vi "Arduino_DigitalRead1.vi"() -> ()   [LabVIEW 2019]
uses:
  <vilib>/LabVIEW Interface for Arduino/Type Defs/Pin Mode.ctl
  <vilib>/LabVIEW Interface for Arduino/Type Defs/Board Type.ctl
  <vilib>/LabVIEW Interface for Arduino/Type Defs/Connection Type.ctl
  <vilib>/LabVIEW Interface for Arduino/LabVIEW Interface for Arduino.lvlib
panel:
  in  "Connection Type (USB/Serial)":T1
  in  "Bytes Per Packet (15)":u32=15
  in  "Board Type (Uno)":T2
  in  "Baud Rate (115200)":u32=115200
  in  "VISA resource":refnum<visa-resource-name>
  out "Value":u8
  out "error close":errorcluster
  out "error read":errorcluster
  in  "stop":bool
  out "error init":errorcluster
  out "error o/i":errorcluster
  in  "Pin Mode (Input)":T3
  in  "Digital I/O Pin":u8
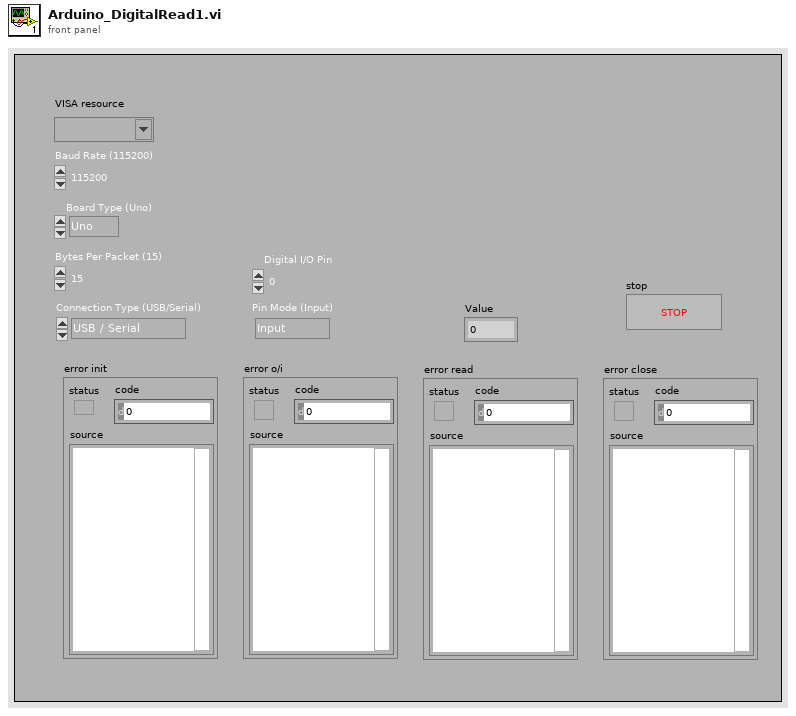
[diagram p1: front panel]
types:
  T1 = typedef "LabVIEW Interface for Arduino.lvlib/Connection Type.ctl" = enum8{"USB / Serial", "XBEE", "BlueSmirf (Bluetooth)"}
  T2 = typedef "LabVIEW Interface for Arduino.lvlib/Board Type.ctl" = enum16{"Uno", "Dimuelanove w/Atmega 328", "Mega 2560"}
  T3 = typedef "LabVIEW Interface for Arduino.lvlib/Pin Mode.ctl" = enum8{"Input", "Output"}
  T4 = typedef "LabVIEW Interface for Arduino.lvlib/Arduino Resource.ctl" = cluster{"VISA resource":refnum<visa-resource-name>, "Board Type":T2, "Connection Type":enum8{"USB / Serial"}, "Bytes Per Packet (15)":u8}
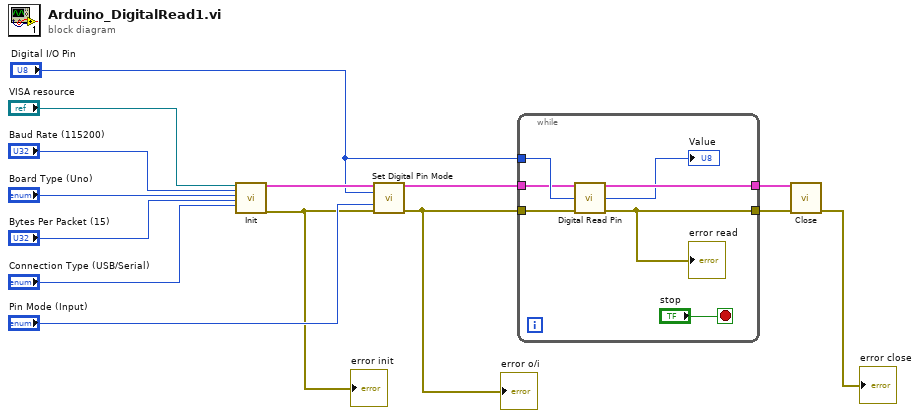
[diagram p0: block diagram]
diagram:
  n1 = call <vilib>:"Init.vi"("VISA resource"="VISA resource", "Baud Rate (115200)"="Baud Rate (115200)", "Board Type (Uno)"="Board Type (Uno)", "Bytes Per Packet (15)"="Bytes Per Packet (15)", "Connection Type (USB/Serial)"="Connection Type (USB/Serial)") -> ("Arduino Resource"=w13:T4, "error out"=w12:errorcluster)  [unwired: 13 in]
  "error init" <- w12
  n2 = call <vilib>:"Set Digital Pin Mode.vi"("Arduino Resource"=w13, "Digital I/O Pin"="Digital I/O Pin", "Pin Mode (Input)"="Pin Mode (Input)", "error in"=w12) -> ("Arduino Resource"=w9:T4, "error out"=w10:errorcluster)  [unwired: 10 in]
  "error o/i" <- w10
  n3 = while {
    tunnel: "Digital I/O Pin" -> [w20]
    tunnel: w10 -> [w19]
    tunnel: w9 -> [w18]
    tunnel: [w17] -> w8
    tunnel: [w16] -> w7
    stop <- "stop" stop-if-true
    n4 = call <vilib>:"Digital Read Pin.vi"("Arduino Resource"=w18, "Digital I/O Pin (0)"=w20, "error in"=w19) -> ("Arduino Resource"=w17:T4, "Value"=→"Value":u8, "error out"=w16:errorcluster)  [unwired: 10 in]
    "error read" <- w16
  }
  n5 = call <vilib>:"Close.vi"("Arduino Resource"=w8, "error in"=w7) -> ("error out"=→"error close":errorcluster)  [unwired: 13 in]
